vi "Read Module Menu Name.vi"(8 "error in":errorcluster, 11 "tag bus configurable plugin editor node in":refnum<class "TEST EDITOR.lvclass">) -> (0 "error out":errorcluster, 2 "Menu Name":string, 3 "tag bus configurable plugin editor node out":refnum<class "TEST EDITOR.lvclass">)   [LabVIEW 2013, in "configuration tests.lvlib" / "TEST EDITOR.lvclass"]
uses:
  TEST EDITOR.lvclass
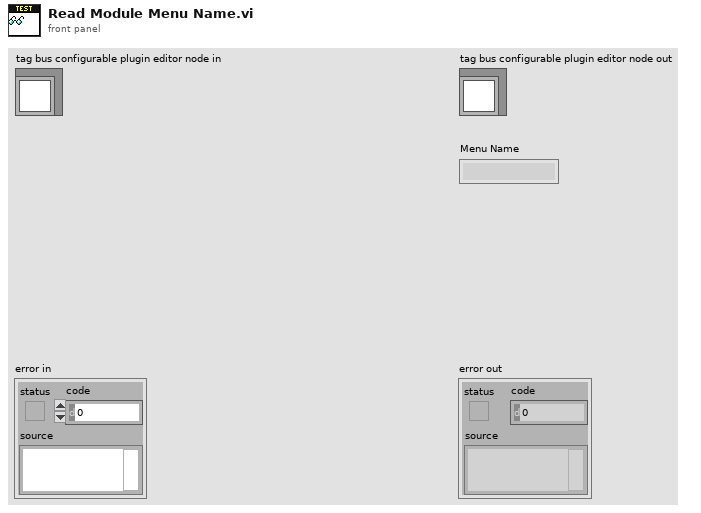
[diagram p1: front panel]
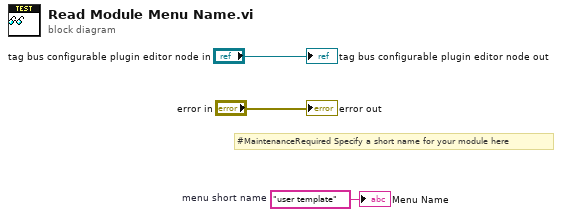
[diagram p0: block diagram]
diagram:
  w1 = "user template"  # menu short name
  # "#MaintenanceRequired Specify a short name for your module here"
  "error out" <- "error in"
  "tag bus configurable plugin editor node out" <- "tag bus configurable plugin editor node in"
  "Menu Name" <- w1
